vi "Set Fields.vi"(8 "error in":errorcluster, 10 "Fields":variant[](array[variant]), 11 "Device Info in":refnum<class "Device Info.lvclass">) -> (0 "error out":errorcluster, 3 "Device Info out":refnum<class "Device Info.lvclass">)   [LabVIEW 2019, in "Electronic Datasheet.lvlib" / "Device Info.lvclass"]
uses:
  Device Info.lvclass
  Device Info.lvclass/Device Info.ctl
  Electronic Datasheet.lvlib
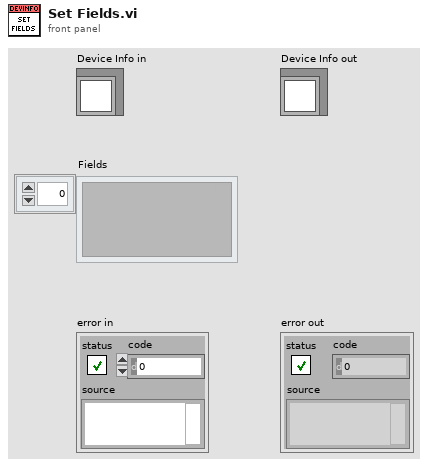
[diagram p1: front panel]
types:
  T1 = cluster{"VendorName":string, "VendorNumber":u32, "ProductName":string, "ProductNumber":u32, "RevisionNumber":u32, "OrderCode":string, "BaudRate_10":bool, "BaudRate_20":bool, "BaudRate_50":bool, "BaudRate_125":bool, "BaudRate_250":bool, "BaudRate_500":bool, "BaudRate_800":bool, "BaudRate_1000":bool, "BaudRate_auto":bool, "SimpleBootUpMaster":bool, "SimpleBootUpSlave":bool, "Granularity":u8, "DynamicChannelsSupported":bool, "CompactPDO":u8, "GroupMessaging":bool, "NrOfRXPDO":u16, "NrOfTXPDO":u16, "LSS_Supported":bool, "LSS_Master":bool, "NG_Slave":bool, "NG_Master":bool, "NrOfNG_MonitoredNodes":u16}
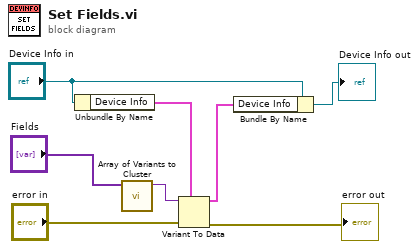
[diagram p0: block diagram]
diagram:
  n1 = Unbundle By Name("Device Info in") -> ("Device Info"=w6:T1)
  n2 = call "Array of Variants to Cluster.vi"("Fields"="Fields") -> ("Variant"=w1:variant)  [unwired: 10 in]
  n3 = Variant To Data(error in="error in", type=w6, Variant=w1) -> (data=w3:T1, error out=→"error out":errorcluster)
  n4 = Bundle By Name(cluster="Device Info in", "Device Info"=w3) -> (→"Device Info out":refnum<class "Device Info.lvclass">)
